vi "Qwand_SIMULINK.vi"(8 "Temperatur [K]":dbl, 9 "Wandtemperatur [K]":dbl=420.0) -> (3 "Qw":dbl)   [LabVIEW 2012]
uses:
  <vilib>/gmath/NI_Gmath.lvlib
panel:
  in  "Zylinderinnenfläche [m^2]":dbl=0.01085
  in  "Wanddicke [m]":dbl=0.1
  in  "Lambda [W*m^-1*K^-1]":dbl[](array[numeric])=[15.0, 16.0, 18.0, 19.0, 21.0, 22.0, 24.0, 25.0, 26.0, 28.0, 29.0]
  in  "Temperaturtabelle [K]":dbl[](array[numeric])=[293.15, 373.15, 473.15, 573.15, 673.15, 773.15, 873.15, 973.15, 1073.15, 1173.15, 1273.15]
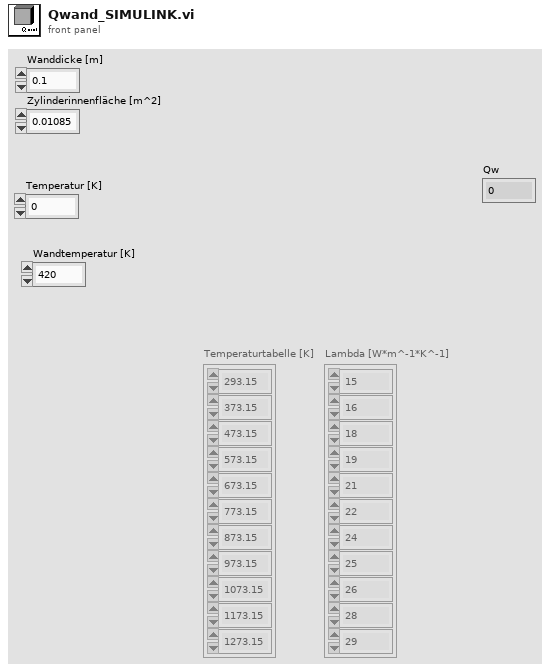
[diagram p1: front panel]
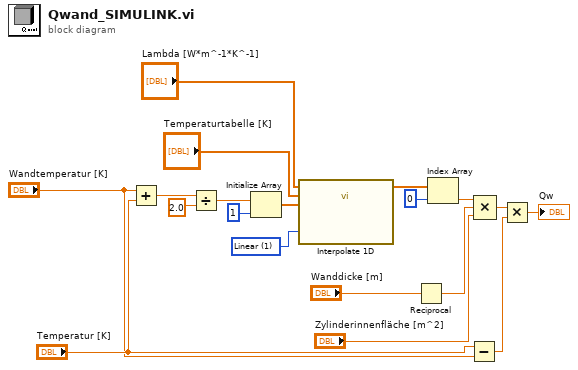
[diagram p0: block diagram]
diagram:
  w19 = 1 items=["Nächste", "Linear", "Spline", "Hermite (kubisch)", "Lagrange"] ("method")
  n1 = Add(x="Wandtemperatur [K]", y="Temperatur [K]") -> (x+y=w8:dbl)
  n2 = Divide(x=w8, y=2.0) -> (x/y=w6:dbl)
  n3 = Initialize Array(w6, 1 ("Dimension")) -> (w16:dbl[])
  n4 = call <vilib>:"Interpolate 1D.vi"("method"=w19, "xi"=w16, "X"="Temperaturtabelle [K]", "Y"="Lambda [W*m^-1*K^-1]") -> ("yi"=w14:dbl[])  [unwired: 5 in, 2 out]
  n5 = Reciprocal(x="Wanddicke [m]") -> (1/x=w9:dbl)
  n6 = Index Array(array=w14, index=0 ("Index")) -> (element=w12:dbl)
  n7 = Subtract(x="Temperatur [K]", y="Wandtemperatur [K]") -> (x-y=w3:dbl)
  n8 = Compound Arithmetic op=MULTIPLY(w12, w9, "Zylinderinnenfläche [m^2]") -> (w2:dbl)
  n9 = Multiply(x=w2, y=w3) -> (x*y=→"Qw":dbl)
